vi "RIB Req - Fuse 5 Test.vi"(0 "Limits File Path":path, 5 "Results File Path":path, 11 "error in":errorcluster) -> (4 "Results Data Array":string[][](array[string]), 15 "error out":errorcluster)   [LabVIEW 2024]
doc: "Template test"
uses:
  <vilib>/addons/_JKI Toolkits/State Machine/_JKI_lib_State_Machine.llb/Select State(s)_err__jki_lib_state_machine.vi
  <vilib>/addons/_JKI Toolkits/State Machine/_JKI_lib_State_Machine.llb/Select State(s)_bool__jki_lib_state_machine.vi
  <vilib>/addons/_JKI Toolkits/State Machine/_JKI_lib_State_Machine.llb/Periodic Trigger__ogtk__JKI-SM__jki_lib_state_machine.vi
  <userlib>/_OpenG.lib/file/file.llb/Strip Path Extension - String__ogtk.vi
  <vilib>/Utility/file.llb/Read Delimited Spreadsheet (string).vi
  <userlib>/_OpenG.lib/file/file.llb/openg_file.lvlib
  <userlib>/_OpenG.lib/appcontrol/appcontrol.llb/openg_application_control.lvlib
  <userlib>/_OpenG.lib/time/time.llb/openg_time.lvlib
  <vilib>/Utility/file.llb/Write Delimited Spreadsheet (string).vi
panel:
  out "Timeout - Test 2":dbl(slide) scale=0.0..5.0
  out "State Test":bool
  in  "Fuse 5 State Error Test":string
  in  "Fuse 5 State Test":string
  in  "Read Start":string
  in  "Read Set":string
  out "Timeout - Test":dbl(slide) scale=0.0..5.0
  out "Fuse 5 Test":bool
  in  "Fuse 5 Error Test":string
  in  "Fuse 5 Test":string
  in  "connection ID":refnum<k16>
  in  "handle out":u64
  in  "Exit":bool
  # "Fuse 5 Test"
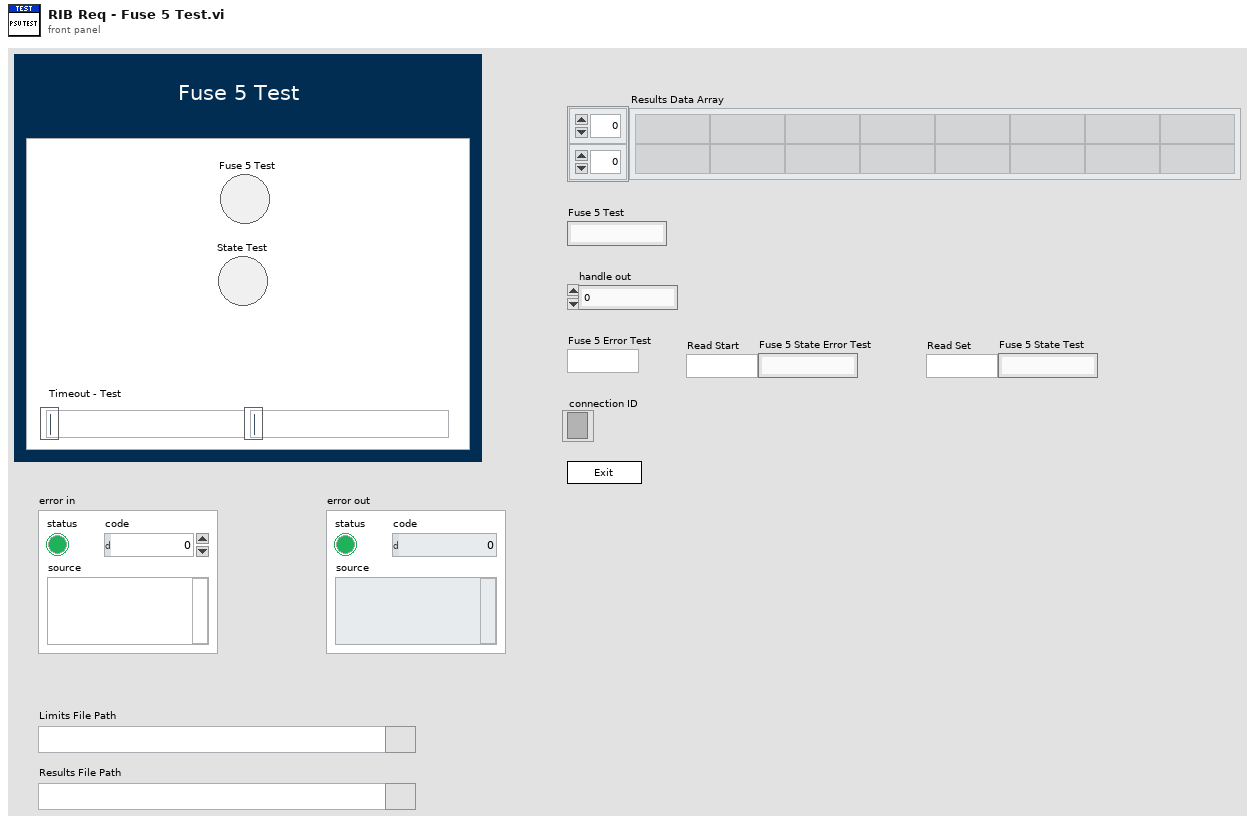
[diagram p1: front panel]
types:
  T1 = enum32{"Invalid", "Standard", "Closed", "Hidden", "Minimized", "Maximized"}
  T2 = enum32{"invalid app kind", "Development System", "Run Time System", "Student Edition", "Embedded LabVIEW", "Evaluation", "Custom"}
  T3 = typedef "FGV - Enum" = enum16{"Cleanup", "Get Data", "Simulator", "Open UDP", "Initialise DAQ", "Initialise I2C"}
  T4 = enum16{"Start Timer", "Get Time", "Pause", "Unpause"}
  T5 = cluster{"Core":cluster{"Current VI Reference":refnum<vi>, "Close Panel on Exit?":bool}, "Limits File Path":path, "Test Limits":string[][], "Results Data Array":string[][], "Results File Path":path, "Voltage":dbl, "connection ID":refnum<k16>, "handle out":u64, "Fuse 5 Test":string, "Fuse 5 Error Test":string, "Read Set":string, "Read Start ":string, "Fuse 5 State Test":string, "Fuse 5 State Error Test":string, "Monitor Test":bool}
  T6 = cluster{"Current VI Reference":refnum<vi>, "Close Panel on Exit?":bool}
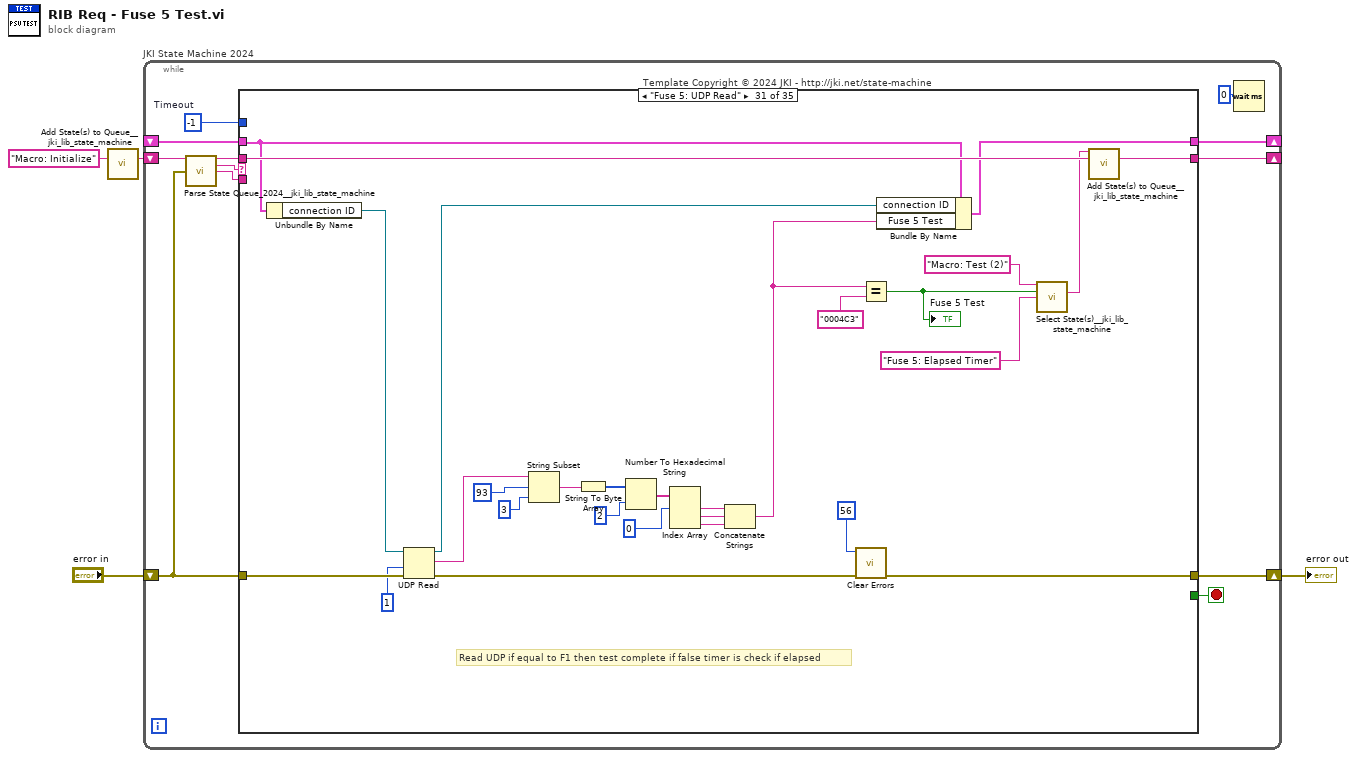
[diagram p0: block diagram]
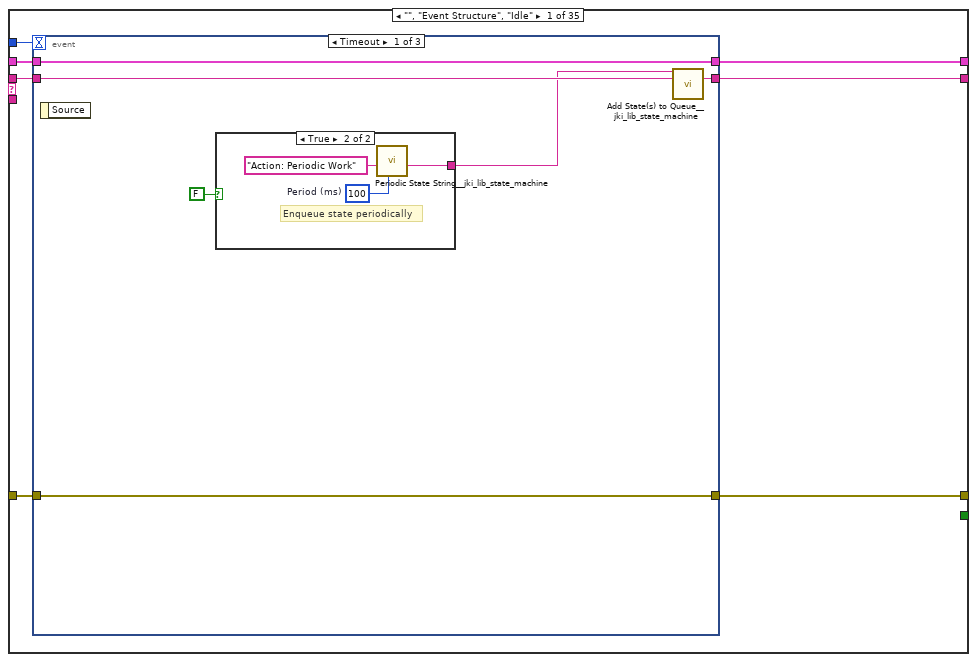
[diagram p2: hidden frame]
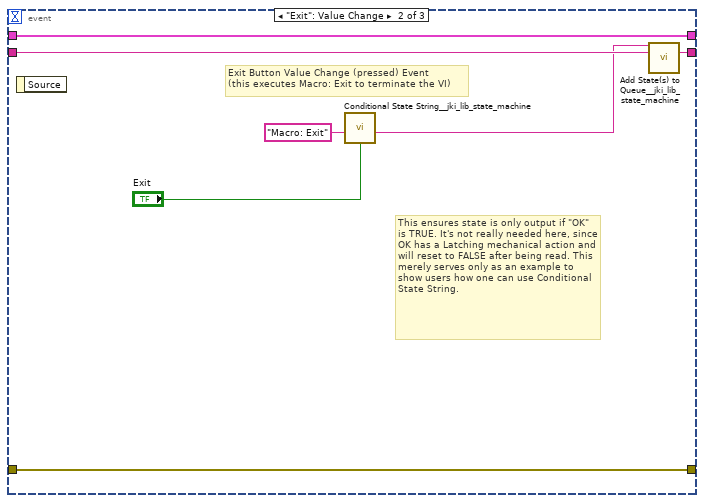
[diagram p4: hidden frame]
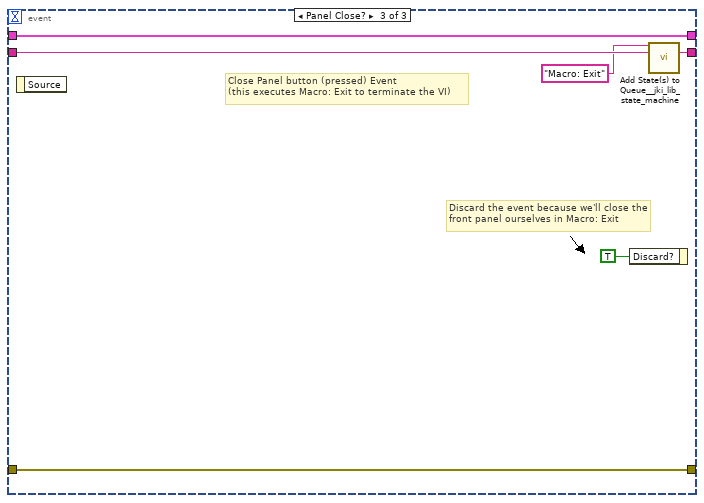
[diagram p5: hidden frame]
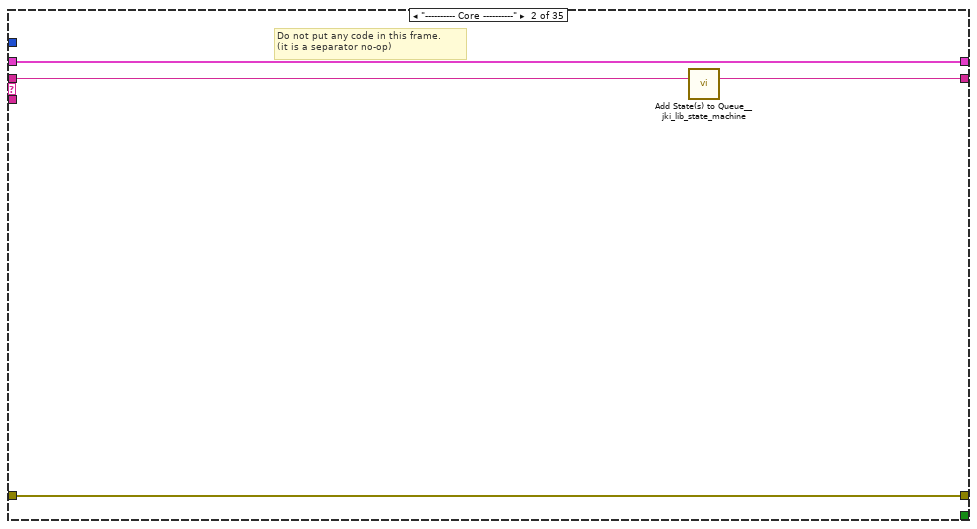
[diagram p6: hidden frame]
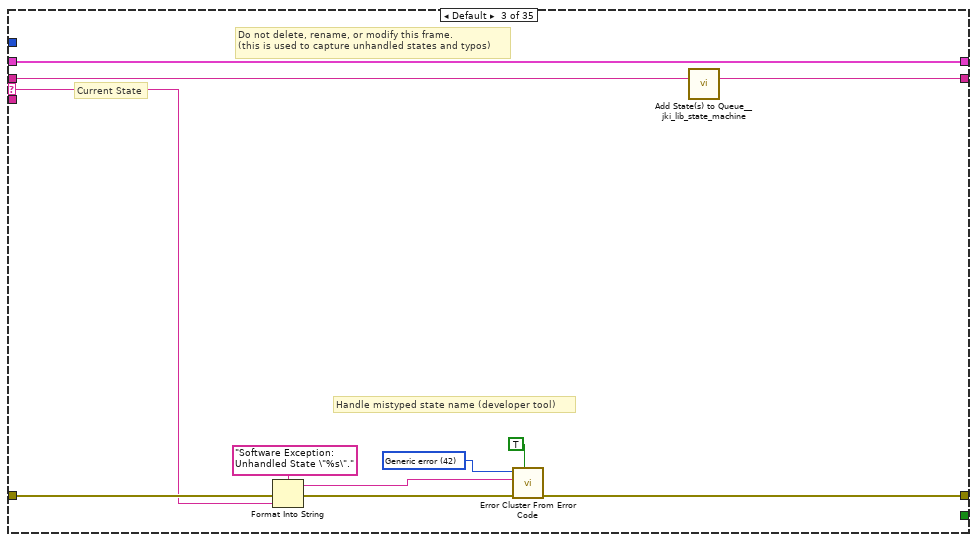
[diagram p7: hidden frame]
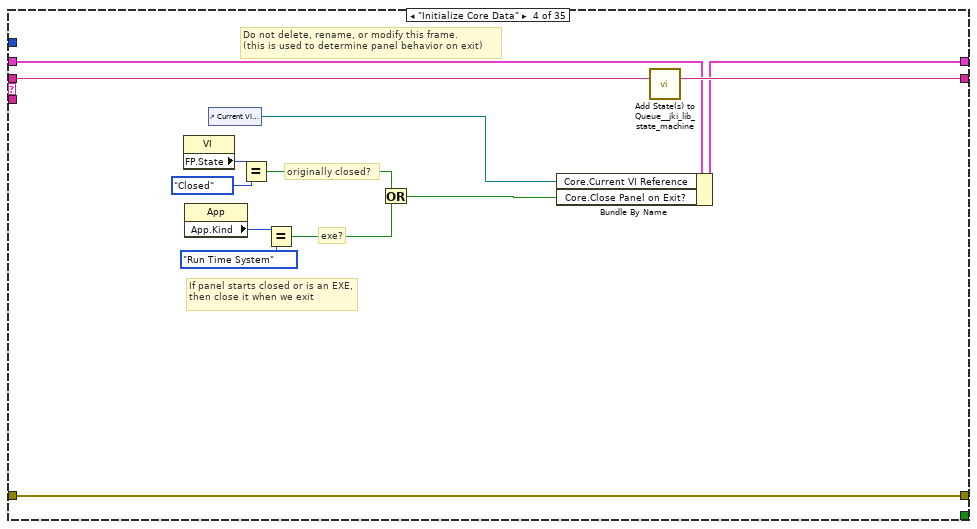
[diagram p8: hidden frame]
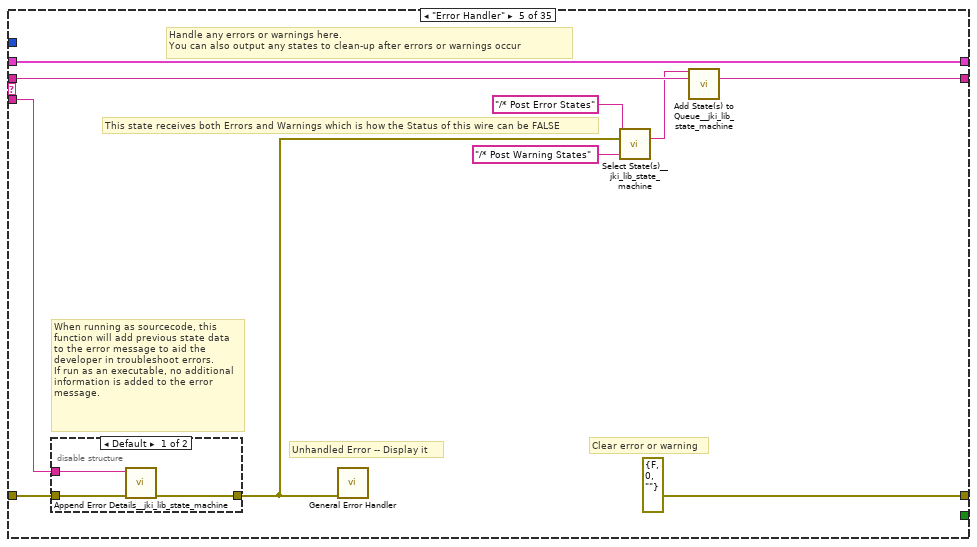
[diagram p9: hidden frame]
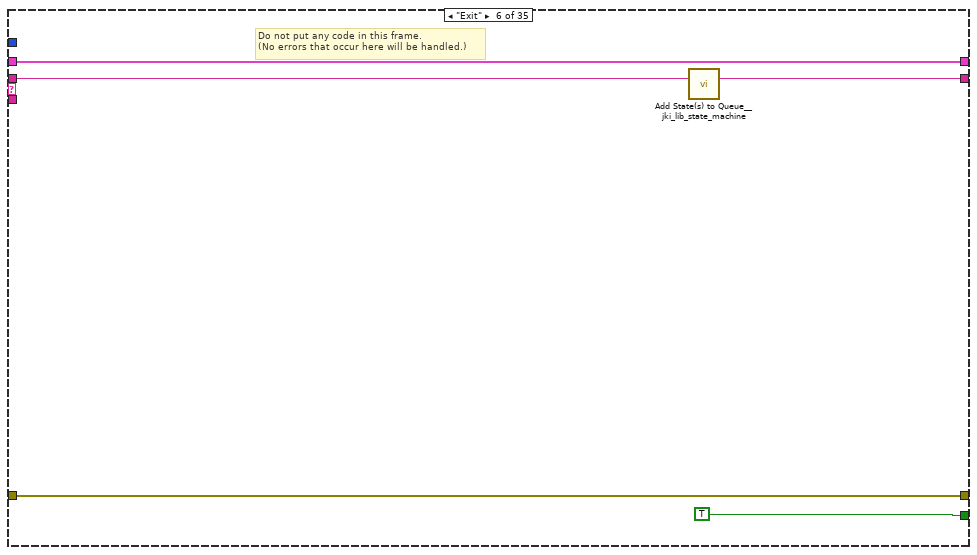
[diagram p11: hidden frame]
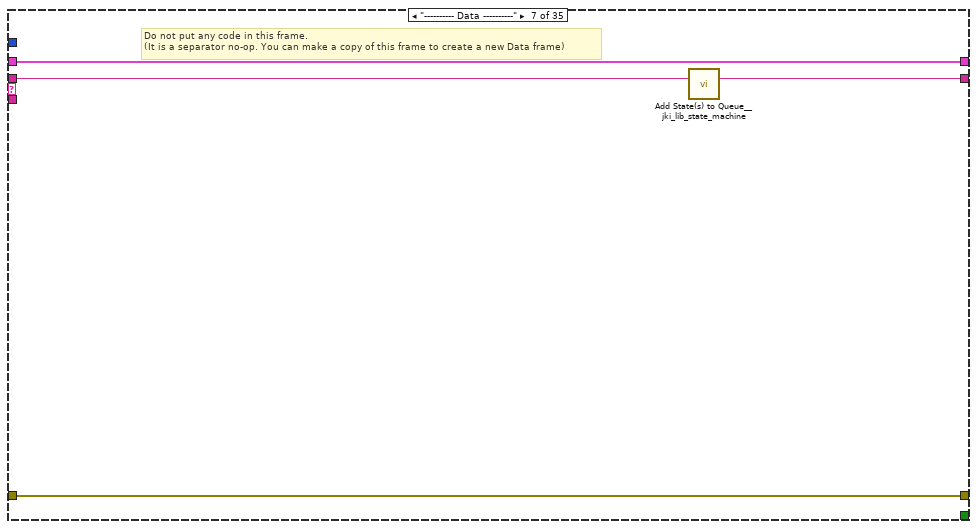
[diagram p12: hidden frame]
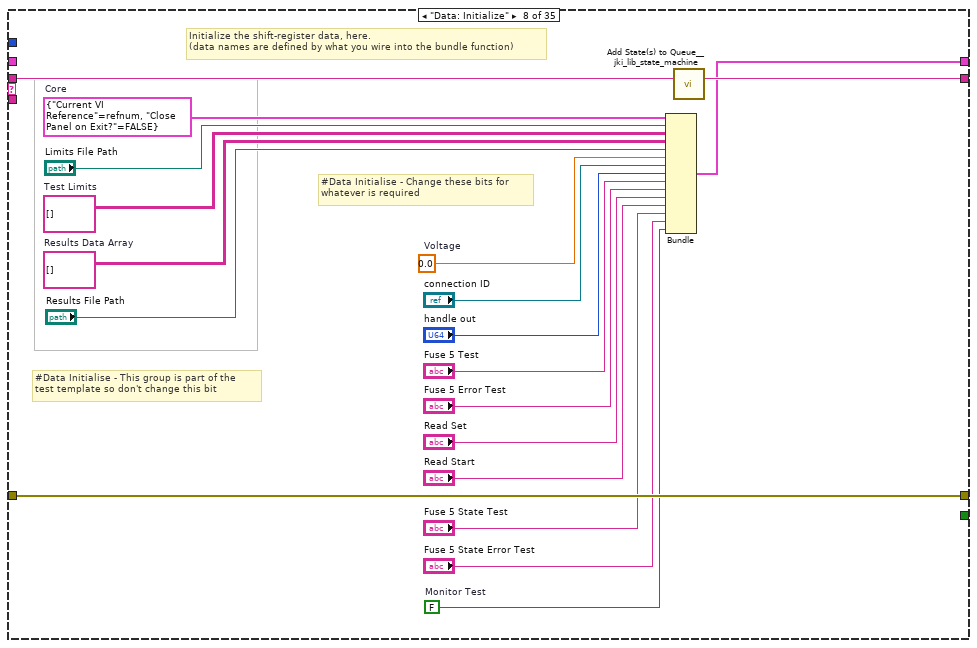
[diagram p13: hidden frame]
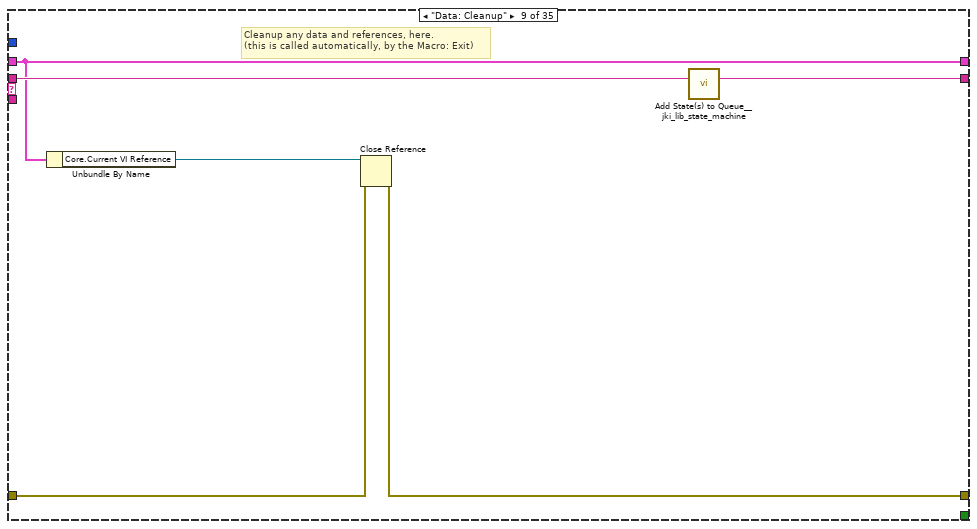
[diagram p14: hidden frame]
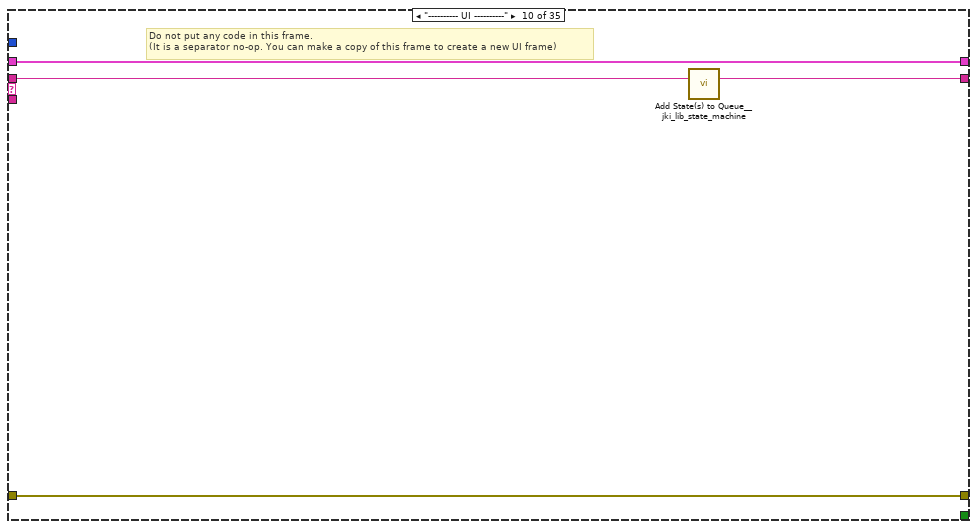
[diagram p15: hidden frame]
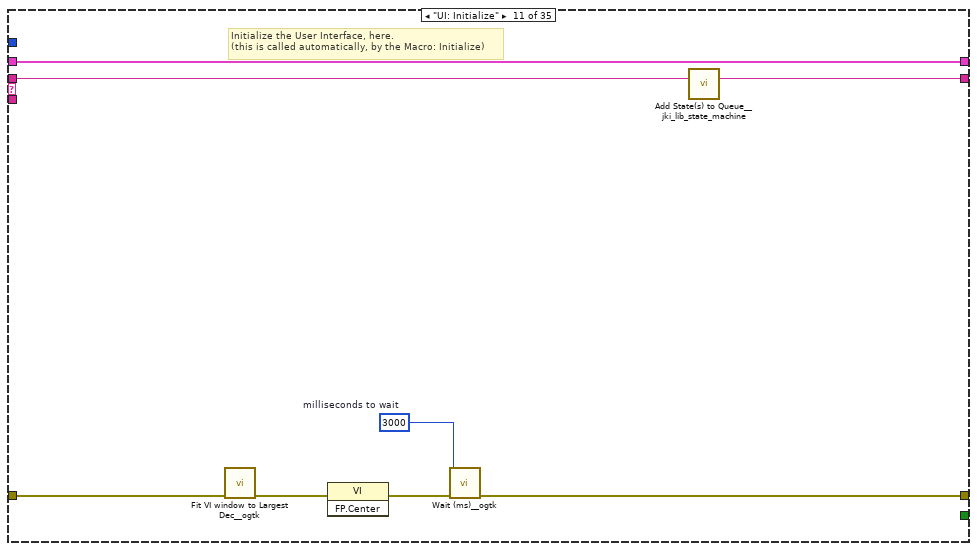
[diagram p16: hidden frame]
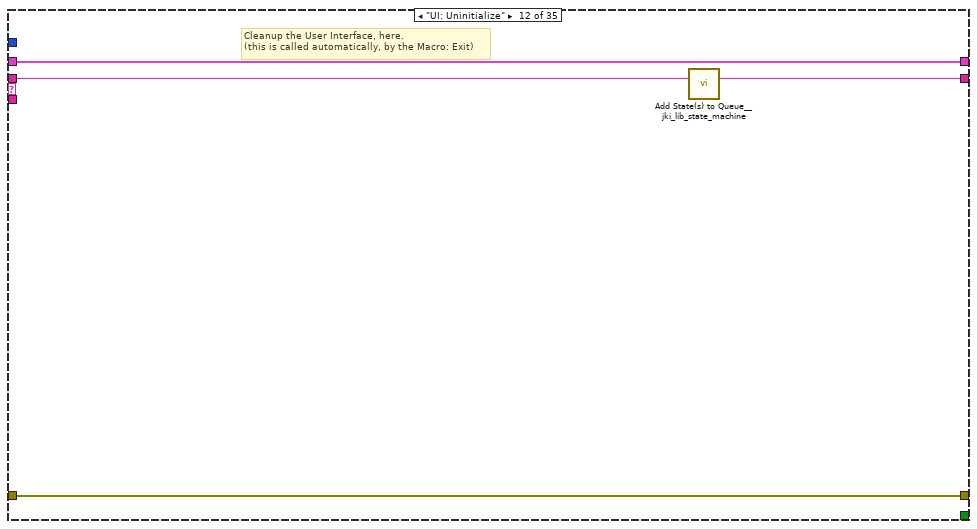
[diagram p17: hidden frame]
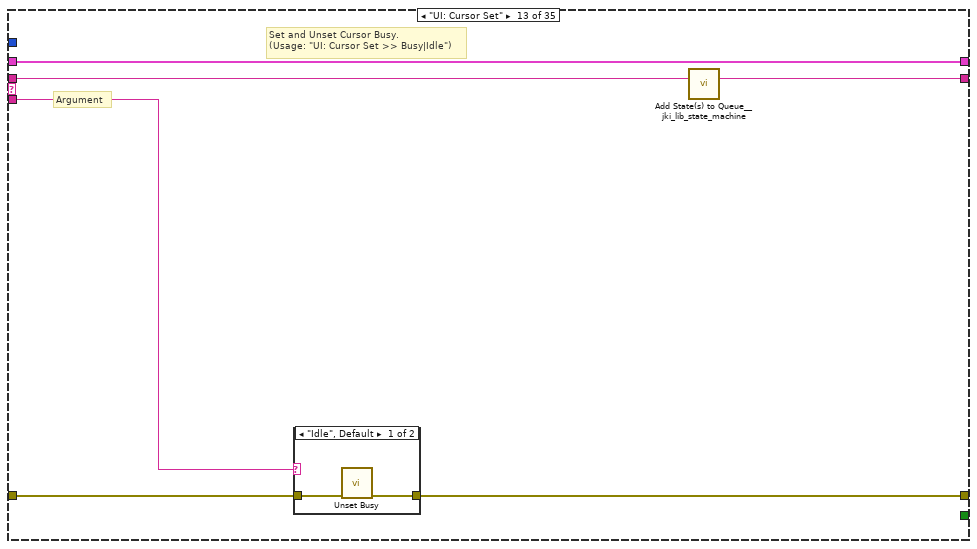
[diagram p18: hidden frame]
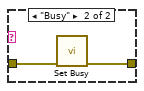
[diagram p19: hidden frame]
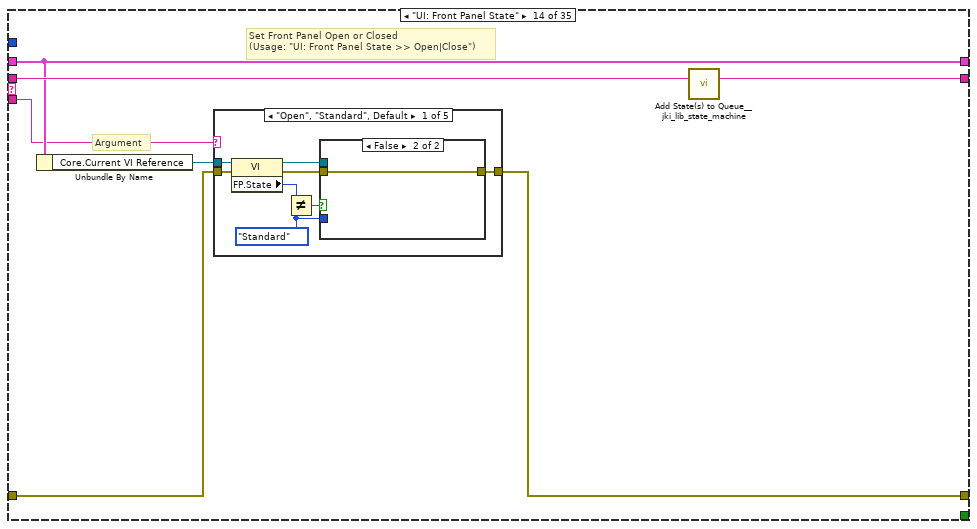
[diagram p20: hidden frame]
diagram:
  n1 = call <vilib>:"Add State(s) to Queue__jki_lib_state_machine.vi"("State(s) in (\"\")"="Macro: Initialize") -> ("States Out"=w4:string)  [unwired: 14 in]
  n2 = while "JKI State Machine 2024" {
    shift-right: [w9] -> _
    shift-left: _ -> [w8]
    shift-right: [w12] -> w1
    shift-left: "error in" -> [w6]
    shift-right: [w11] -> _
    shift-left: w4 -> [w13]
    stop <- w10 stop-if-true
    w7 = -1  # Timeout
    # "Template Copyright © 2024 JKI - http://jki.net/state-machine"
    n3 = call <vilib>:"Parse State Queue_2024__jki_lib_state_machine.vi"("State Queue"=w13, "Error In (no error)"=w6) -> ("Remaining States"=w15:string, "Current State"=w16:string, "Arguments"=w14:string)  [unwired: 11 in]
    n4 = case shown="\"Fuse 5: UDP Read\"" w16 {
      selector: w16 -> [_ _ w50 _ _ _ _ _ _ _ _ _ _ _ _ _ _ _ _ _ _ _ _ _ _ _ _ _ _ _ _ _ _ _ _]
      tunnel: w15 -> [w23 w49 w54 w73 w83 w92 w96 w115 w121 w125 w133 w137 w143 w154 w223 w228 w233 w238 w243 w252 w256 w269 w286 w299 w303 w312 w316 w325 w335 w344 w372 w384 w394 w418 w430]
      tunnel: w14 -> [_ _ _ _ w78 _ _ _ _ _ _ _ w138 w148 _ _ _ _ _ _ _ _ _ _ _ _ _ _ _ _ _ _ _ _ _]
      tunnel: w8 -> [w21 w46 w52 w66 w80 w90 w93 _ w116 w122 w131 w135 w141 w150 w220 w225 w230 w235 w240 w250 w253 w259 w278 w291 w300 w308 w313 w323 w333 w342 w356 w382 w392 w405 w428]
      tunnel: [w20 w47 w56 w70 errorcluster {"status"=FALSE, "code"=0, "source"=""} ("error out") w89 w94 w112 w117 w123 w129 w134 w139 w151 w221 w226 w231 w236 w241 w247 w254 w265 w283 w296 w301 w310 w314 w320 w326 w339 w354 w376 w385 w403 w422] -> w12
      tunnel: w6 -> [w17 w47 w55 w70 w79 w89 w94 w112 w118 w123 w130 w134 w140 w152 w221 w226 w231 w236 w241 w247 w254 w264 w282 w295 w301 w309 w314 w321 w327 w340 w357 w377 w386 w399 w423]
      tunnel: [w22 w48 w53 w72 w82 w91 w95 w114 w120 w124 w132 w136 w142 w153 w222 w227 w232 w237 w242 w251 w255 w268 w285 w298 w302 w311 w315 w324 w334 w343 w371 w383 w393 w417 w429] -> w11
      tunnel: [_ _ _ _ _ TRUE _ _ _ _ _ _ _ _ _ _ _ _ _ _ _ _ _ _ _ _ _ _ _ _ _ _ _ _ _] -> w10
      tunnel: [w19 w46 w52 w71 w80 w90 w93 w113 w116 w122 w131 w135 w141 w150 w220 w225 w230 w235 w240 w250 w253 w258 w277 w290 w300 w308 w313 w322 w333 w341 w370 w382 w392 w416 w428] -> w9
      tunnel: w7 -> [w18 _ _ _ _ _ _ _ _ _ _ _ _ _ _ _ _ _ _ _ _ _ _ _ _ _ _ _ _ _ _ _ _ _ _]
      frame "", "Event Structure", "Idle" {
        n5 = event shown="[0] Timeout" {
          selector: _ -> [_ _ _]
          dyn-events: _ -> [_ _ _]
          timeout: w18 -> [_ _ _]
          tunnel: w23 -> [w29 w39 w45]
          tunnel: [w28 w38 w44] -> w22
          tunnel: w21 -> [w26 w36 w42]
          tunnel: [w27 w37 w43] -> w20
          tunnel: w17 -> [w27 w37 w43]
          tunnel: [w26 w36 w42] -> w19
          event Timeout {
            n6 = event-data() -> ()  [unwired: 1 in, 1 out]
            n7 = case shown="True" FALSE {
              tunnel: [_ w32] -> w25
              frame False {
              }
              frame True {
                w30 = u32 100  # Period (ms)
                # "Enqueue state periodically"
                n8 = call <vilib>:"Periodic State String__jki_lib_state_machine.vi"("Period (ms)"=w30, "State"="Action: Periodic Work") -> ("State Out"=w32:string)  [unwired: 9 in]
              }
            }
            n9 = call <vilib>:"Add State(s) to Queue__jki_lib_state_machine.vi"("State(s) in Front (\"\")"=w25, "State(s) in (\"\")"=w29) -> ("States Out"=w28:string)  [unwired: 13 in]
          }
          event "Exit": Value Change {
            # "This ensures state is only output if \"OK\" is TRUE. It's not really needed here, since OK has a Latching mechanical action and will reset to FALSE after being read. This merely serves only as an example to show users how one can use Conditional State String."
            # "Exit Button Value Change (pressed) Event\n(this executes Macro: Exit to terminate the VI)"
            n10 = event-data() -> ()  [unwired: 1 in, 1 out]
            n11 = call <vilib>:"Conditional State String__jki_lib_state_machine.vi"("Do State(s)?"="Exit", "State"="Macro: Exit") -> ("State Out"=w33:string)  [unwired: 7 in]
            n12 = call <vilib>:"Add State(s) to Queue__jki_lib_state_machine.vi"("State(s) in Front (\"\")"=w33, "State(s) in (\"\")"=w39) -> ("States Out"=w38:string)  [unwired: 13 in]
          }
          event Panel Close? {
            # "Discard the event because we'll close the front panel ourselves in Macro: Exit"
            # "Close Panel button (pressed) Event\n(this executes Macro: Exit to terminate the VI)"
            n13 = event-data() -> ()  [unwired: 1 in, 1 out]
            n14 = event-data("Discard?"=TRUE) -> ()  [unwired: 1 in, 1 out]
            n15 = call <vilib>:"Add State(s) to Queue__jki_lib_state_machine.vi"("State(s) in Front (\"\")"="Macro: Exit", "State(s) in (\"\")"=w45) -> ("States Out"=w44:string)  [unwired: 13 in]
          }
        }
      }
      frame "---------- Core ----------" {
        # "Do not put any code in this frame.\n(it is a separator no-op)"
        n16 = call <vilib>:"Add State(s) to Queue__jki_lib_state_machine.vi"("State(s) in (\"\")"=w49) -> ("States Out"=w48:string)  [unwired: 14 in]
      }
      frame Default {
        w59 = 42 items=["No error", "Argument error", "Memory is full", "Out of zone", "End of file", "File already open", "Generic file I/O error", "File not found", "File permission error", "Disk is full", "Duplicate path", "Too many files open", "System feature not enabled", "Resource file not found", "Cannot add resource", "Resource not found", "Image not found", "Image memory error", "Pen does not exist", "Config type invalid", "Config token not found", "Config parse error", "Config memory error", "Bad external code format", "Bad external code offset", "External code not present", "Null window", "Destroy window error", "Null menu", "Print aborted", "Bad print record", "Print driver error", "Windows error during printing", "Memory error during printing", "Print dialog error", "Generic print error", "Invalid device refnum", "Device not found", "Device parameter error", "Device unit error", "Cannot open device", "Device call aborted", "Generic error", "Cancelled by user", "Object ID too low", "Object ID too high", "Object not in heap", "Unknown heap", "Unknown object (invalid DefProc)", "Unknown object (DefProc not in table)", "Message out of range", "Invalid (null) method", "Unknown message", "Manager call not supported", "Bad address", "Network operation in progress", "Network operation timed out", "Connection is busy", "Network attribute not supported", "Network error", "Address in use", "System out of memory", "Connection aborted", "Connection refused", "Not connected", "Already connected", "Connection closed", "Initialization error (interapplication manager)", "Bad occurrence", "Wait on unbound occurrence handler", "Occurrence queue overflow", "Datalog type conflict", "Unused", "Unrecognized type (interapplication manager)", "Memory corrupt", "Failed to make temporary DLL", "Old CIN version", "Drag socket not found", "Failed to load drop-object", "Failed to register OLE object", "Failed to release OLE object", "Format specifier type mismatch", "Unknown format specifier", "Too few format specifiers", "Too many format specifiers", "Scan failed", "Newer CIN version", "Error converting to variant", "Runtime menu error", "Password tampered", "Variant attribute not found", "Incompatible variant data type", "Event data is not available", "Event Store is not present", "Occurrence is not found", "Event Queue is not created", "Event info is not available", "Refnum passed is NULL", "Error retrieving Class GUID", "Error retrieving CoClass GUID", "Error retrieving TypeLib GUID.", "Bad built application magic bytes.", "Specific driver is different from the specific driver associated with the Logical Name.", "There is no session opened to the class driver.", "Max Error", "MAX - Error with config objects", "MAX - Error loading configuration", "MAX - Group not supported"]
        # "Current State"
        # "Do not delete, rename, or modify this frame.\n(this is used to capture unhandled states and typos)"
        # "Handle mistyped state name (developer tool)"
        n17 = Format Into String(format string="Software Exception: Unhandled State \"%s\"." ("message"), error in=w55, w50) -> (resulting string=w58:string, error out=w57:errorcluster)  [unwired: 1 in]
        n18 = call <vilib>:"Error Cluster From Error Code.vi"("show call chain? (False)"=TRUE, "error in (no error)"=w57, "error message (\"\")"=w58, "error code (0)"=w59) -> ("error out"=w56:errorcluster)  [unwired: 5 in]
        n19 = call <vilib>:"Add State(s) to Queue__jki_lib_state_machine.vi"("State(s) in (\"\")"=w54) -> ("States Out"=w53:string)  [unwired: 14 in]
      }
      frame "Initialize Core Data" {
        # "Do not delete, rename, or modify this frame.\n(this is used to determine panel behavior on exit)"
        # "originally closed?"
        # "exe?"
        # "If panel starts closed or is an EXE, then close it when we exit"
        n20 = property class="VI"() -> ("FP.State"=w63:T1)  [unwired: 2 in, 2 out]
        n21 = property class="App"() -> ("App.Kind"=w69:T2)  [unwired: 2 in, 2 out]
        n22 = control-ref of="Current VI Reference"() -> (w64:refnum<vi>)
        n23 = Equal?(x=w63, y=T1."Closed" ("Front Panel Window:State")) -> (x = y?=w61:bool)
        n24 = Equal?(x=w69, y=T2."Run Time System" ("Application:Kind")) -> (x = y?=w67:bool)
        n25 = Or(x=w61, y=w67) -> (x .or. y?=w65:bool)
        n26 = Bundle By Name(cluster=w66, "Core.Current VI Reference"=w64, "Core.Close Panel on Exit?"=w65) -> (w71:T5)
        n27 = call <vilib>:"Add State(s) to Queue__jki_lib_state_machine.vi"("State(s) in (\"\")"=w73) -> ("States Out"=w72:string)  [unwired: 14 in]
      }
      frame "Error Handler" {
        # "When running as sourcecode, this function will add previous state data to the error message to aid the developer in troubleshoot errors.\nIf run as an executable, no additional information is added to the error message."
        # "This state receives both Errors and Warnings which is how the Status of this wire can be FALSE"
        # "Unhandled Error -- Display it"
        # "Handle any errors or warnings here.\nYou can also output any states to clean-up after errors or warnings occur"
        # "Clear error or warning"
        n28 = disable-structure shown="Default" {
          disable-tunnel: w79 -> [w86 w87]
          disable-tunnel: w78 -> [w85 _]
          disable-tunnel: [w84 w87] -> w77
          frame condition #0 (active) {
            n29 = call <vilib>:"Append Error Details__jki_lib_state_machine.vi"("error in (no error)"=w86, "Previous State and Argument(s)"=w85) -> ("error out"=w84:errorcluster)  [unwired: 9 in]
          }
          frame condition #1 {
          }
        }
        n30 = call <vilib>:"General Error Handler.vi"("error in (no error)"=w77) -> ()  [unwired: 10 in, 5 out]
        n31 = call-poly <vilib>:"Select State(s)__jki_lib_state_machine.vi"("State(s) if True (\"\")"="/* Post Error States", "Select"=w77, "State(s) if False (\"\")"="/* Post Warning States") -> ("States Out"=w75:string)  [unwired: 12 in]
        n32 = call <vilib>:"Add State(s) to Queue__jki_lib_state_machine.vi"("State(s) in Front (\"\")"=w75, "State(s) in (\"\")"=w83) -> ("States Out"=w82:string)  [unwired: 13 in]
      }
      frame "Exit" {
        # "Do not put any code in this frame.\n(No errors that occur here will be handled.)"
        n33 = call <vilib>:"Add State(s) to Queue__jki_lib_state_machine.vi"("State(s) in (\"\")"=w92) -> ("States Out"=w91:string)  [unwired: 14 in]
      }
      frame "---------- Data ----------" {
        # "Do not put any code in this frame.\n(It is a separator no-op. You can make a copy of this frame to create a new Data frame)"
        n34 = call <vilib>:"Add State(s) to Queue__jki_lib_state_machine.vi"("State(s) in (\"\")"=w96) -> ("States Out"=w95:string)  [unwired: 14 in]
      }
      frame "Data: Initialize" {
        w97 = FALSE  # Monitor Test
        w106 = 0.0  # Voltage
        w108 = string[][] []  # Results Data Array
        w109 = string[][] []  # Test Limits
        w111 = T6 {"Current VI Reference"=refnum, "Close Panel on Exit?"=FALSE}  # Core
        # "#Data Initialise - Change these bits for\nwhatever is required"
        # "#Data Initialise - This group is part of the\ntest template so don't change this bit"
        # "Initialize the shift-register data, here.\n(data names are defined by what you wire into the bundle function)"
        n35 = Bundle("Core"=w111, "Limits File Path"="Limits File Path", "Test Limits"=w109, "Results Data Array"=w108, "Results File Path"="Results File Path", "Voltage"=w106, "connection ID"="connection ID", "handle out"="handle out", "Fuse 5 Test"="Fuse 5 Test", "Fuse 5 Error Test"="Fuse 5 Error Test", "Read Set"="Read Set", "Read Start"="Read Start", "Fuse 5 State Test"="Fuse 5 State Test", "Fuse 5 State Error Test"="Fuse 5 State Error Test", "Monitor Test"=w97) -> (w113:T5)  [unwired: 1 in]
        n36 = call <vilib>:"Add State(s) to Queue__jki_lib_state_machine.vi"("State(s) in (\"\")"=w115) -> ("States Out"=w114:string)  [unwired: 14 in]
      }
      frame "Data: Cleanup" {
        # "Cleanup any data and references, here.\n(this is called automatically, by the Macro: Exit)"
        n37 = Unbundle By Name(w116) -> ("Core.Current VI Reference"=w119:refnum<vi>)
        n38 = Close Reference(reference=w119, error in (no error)=w118) -> (error out=w117:errorcluster)
        n39 = call <vilib>:"Add State(s) to Queue__jki_lib_state_machine.vi"("State(s) in (\"\")"=w121) -> ("States Out"=w120:string)  [unwired: 14 in]
      }
      frame "---------- UI ----------" {
        # "Do not put any code in this frame.\n(It is a separator no-op. You can make a copy of this frame to create a new UI frame)"
        n40 = call <vilib>:"Add State(s) to Queue__jki_lib_state_machine.vi"("State(s) in (\"\")"=w125) -> ("States Out"=w124:string)  [unwired: 14 in]
      }
      frame "UI: Initialize" {
        w128 = u32 3000  # milliseconds to wait
        # "Initialize the User Interface, here.\n(this is called automatically, by the Macro: Initialize)"
        n41 = call <userlib>:"Fit VI window to Largest Dec__ogtk.vi"("error in (no error)"=w130) -> ("error out"=w126:errorcluster)  [unwired: 5 in, 1 out]
        n42 = invoke class="VI" method="FP.Center"(error in=w126) -> (error out=w127:errorcluster)  [unwired: 2 in, 2 out]
        n43 = call <userlib>:"Wait (ms)__ogtk.vi"("error in (no error)"=w127, "milliseconds to wait"=w128) -> ("error out"=w129:errorcluster)  [unwired: 8 in, 1 out]
        n44 = call <vilib>:"Add State(s) to Queue__jki_lib_state_machine.vi"("State(s) in (\"\")"=w133) -> ("States Out"=w132:string)  [unwired: 14 in]
      }
      frame "UI: Uninitialize" {
        # "Cleanup the User Interface, here.\n(this is called automatically, by the Macro: Exit)"
        n45 = call <vilib>:"Add State(s) to Queue__jki_lib_state_machine.vi"("State(s) in (\"\")"=w137) -> ("States Out"=w136:string)  [unwired: 14 in]
      }
      frame "UI: Cursor Set" {
        # "Argument"
        # "Set and Unset Cursor Busy.\n(Usage: \"UI: Cursor Set >> Busy|Idle\")"
        n46 = case shown="\"Idle\", Default" w138 {
          tunnel: w140 -> [w145 w147]
          tunnel: [w144 w146] -> w139
          frame "Idle", Default {
            n47 = call <vilib>:"Unset Busy.vi"("error in (no error)"=w145) -> ("error out"=w144:errorcluster)  [unwired: 10 in]
          }
          frame "Busy" {
            n48 = call <vilib>:"Set Busy.vi"("error in (no error)"=w147) -> ("error out"=w146:errorcluster)  [unwired: 9 in, 1 out]
          }
        }
        n49 = call <vilib>:"Add State(s) to Queue__jki_lib_state_machine.vi"("State(s) in (\"\")"=w143) -> ("States Out"=w142:string)  [unwired: 14 in]
      }
      frame "UI: Front Panel State" {
        # "Argument"
        # "Set Front Panel Open or Closed\n(Usage: \"UI: Front Panel State >> Open|Close\")"
        n50 = Unbundle By Name(w150) -> ("Core.Current VI Reference"=w149:refnum<vi>)
        n51 = case shown="\"Open\", \"Standard\", Default" w148 {
          tunnel: w152 -> [w160 w175 w186 w199 w212]
          tunnel: [w162 w176 w188 w201 w214] -> w151
          tunnel: w149 -> [w161 w173 w187 w200 w213]
          frame "Open", "Standard", Default {
            w155 = T1."Standard" ("State")
            n52 = property class="VI"(reference=w161, error in=w160) -> (reference out=w158:refnum<vi>, error out=w159:errorcluster, "FP.State"=w157:T1)
            n53 = Not Equal?(x=w157, y=w155) -> (x != y?=w156:bool)
            n54 = case shown="False" w156 {
              tunnel: [w166 w168] -> w162
              tunnel: w159 -> [w165 w168]
              tunnel: w158 -> [w164 _]
              tunnel: w155 -> [w163 _]
              frame True {
                n55 = invoke class="VI" method="FP.Open"(reference=w164, error in=w165, "Activate"=TRUE, "State"=w163) -> (error out=w166:errorcluster)  [unwired: 1 in, 4 out]
              }
              frame False {
              }
            }
          }
          frame "Close", "Closed" {
            n56 = property class="VI"(reference=w173, error in=w175) -> (reference out=w172:refnum<vi>, error out=w174:errorcluster, "FP.State"=w170:T1)
            n57 = Not Equal?(x=w170, y=T1."Closed" ("Front Panel Window:State")) -> (x != y?=w169:bool)
            n58 = case shown="True" w169 {
              tunnel: [w177 w180] -> w176
              tunnel: w174 -> [w177 w179]
              tunnel: w172 -> [_ w178]
              frame False {
              }
              frame True {
                n59 = invoke class="VI" method="FP.Close"(reference=w178, error in=w179) -> (error out=w180:errorcluster)  [unwired: 1 in, 2 out]
              }
            }
          }
          frame "Hidden", "Hide" {
            w181 = T1."Hidden" ("State")
            n60 = property class="VI"(reference=w187, error in=w186) -> (reference out=w184:refnum<vi>, error out=w185:errorcluster, "FP.State"=w183:T1)
            n61 = Not Equal?(x=w183, y=w181) -> (x != y?=w182:bool)
            n62 = case shown="True" w182 {
              tunnel: [w192 w193] -> w188
              tunnel: w185 -> [w191 w193]
              tunnel: w184 -> [w190 _]
              tunnel: w181 -> [w189 _]
              frame True {
                n63 = invoke class="VI" method="FP.Open"(reference=w190, error in=w191, "State"=w189) -> (error out=w192:errorcluster)  [unwired: 2 in, 4 out]
              }
              frame False {
              }
            }
          }
          frame "Minimize", "Minimized" {
            w194 = T1."Minimized" ("State")
            n64 = property class="VI"(reference=w200, error in=w199) -> (reference out=w197:refnum<vi>, error out=w198:errorcluster, "FP.State"=w196:T1)
            n65 = Not Equal?(x=w196, y=w194) -> (x != y?=w195:bool)
            n66 = case shown="True" w195 {
              tunnel: [w205 w206] -> w201
              tunnel: w198 -> [w204 w206]
              tunnel: w197 -> [w203 _]
              tunnel: w194 -> [w202 _]
              frame True {
                n67 = invoke class="VI" method="FP.Open"(reference=w203, error in=w204, "State"=w202) -> (error out=w205:errorcluster)  [unwired: 2 in, 4 out]
              }
              frame False {
              }
            }
          }
          frame "Maximize", "Maximized" {
            w207 = T1."Maximized" ("State")
            n68 = property class="VI"(reference=w213, error in=w212) -> (reference out=w210:refnum<vi>, error out=w211:errorcluster, "FP.State"=w209:T1)
            n69 = Not Equal?(x=w209, y=w207) -> (x != y?=w208:bool)
            n70 = case shown="True" w208 {
              tunnel: [w218 w219] -> w214
              tunnel: w211 -> [w217 w219]
              tunnel: w210 -> [w216 _]
              tunnel: w207 -> [w215 _]
              frame True {
                n71 = invoke class="VI" method="FP.Open"(reference=w216, error in=w217, "State"=w215) -> (error out=w218:errorcluster)  [unwired: 2 in, 4 out]
              }
              frame False {
              }
            }
          }
        }
        n72 = call <vilib>:"Add State(s) to Queue__jki_lib_state_machine.vi"("State(s) in (\"\")"=w154) -> ("States Out"=w153:string)  [unwired: 14 in]
      }
      frame "---------- Macro ----------" {
        # "Do not put any code in this frame.\n(It is a separator no-op. You can make a copy of this frame to create a new Macro frame)"
        n73 = call <vilib>:"Add State(s) to Queue__jki_lib_state_machine.vi"("State(s) in (\"\")"=w223) -> ("States Out"=w222:string)  [unwired: 14 in]
      }
      frame "Macro: Initialize" {
        # "Initialization Macro\n(This is called once, when the VI starts)"
        n74 = call <vilib>:"Add State(s) to Queue__jki_lib_state_machine.vi"("State(s) in Front (\"\")"="Data: Initialize\nInitialize Core Data\nUI: Initialize\nUI: Front Panel State >> Open\nFuse 5: Initialise\nMacro: Test", "State(s) in (\"\")"=w228) -> ("States Out"=w227:string)  [unwired: 13 in]
      }
      frame "Macro: Test" {
        # "#Test Macro - Add the sequence \nfor measurments and limits testing here"
        n75 = call <vilib>:"Add State(s) to Queue__jki_lib_state_machine.vi"("State(s) in Front (\"\")"="Limits Test: Read Limits File\nFuse 5: Initialise\nFuse 5: Start Timer\nFuse 5: I2C Measurment\nFuse 5: UDP Read", "State(s) in (\"\")"=w233) -> ("States Out"=w232:string)  [unwired: 13 in]
      }
      frame "Macro: Test (2)" {
        # "#Test Macro - Add the sequence \nfor measurments and limits testing here"
        n76 = call <vilib>:"Add State(s) to Queue__jki_lib_state_machine.vi"("State(s) in Front (\"\")"="Fuse 5: Start Timer (State)\nFuse 5: UDP Read (State)", "State(s) in (\"\")"=w238) -> ("States Out"=w237:string)  [unwired: 13 in]
      }
      frame "Macro: Limits" {
        # "Do not put any code in this frame.\n(It is a separator no-op. You can make a copy of this frame to create a new Macro frame)"
        n77 = call <vilib>:"Add State(s) to Queue__jki_lib_state_machine.vi"("State(s) in Front (\"\")"="Limits Test: Fuse 5 Test\nLimits Test: Fuse 5 State Test\nResults Data: Write Results Data\nMacro: Exit", "State(s) in (\"\")"=w243) -> ("States Out"=w242:string)  [unwired: 13 in]
      }
      frame "Macro: Exit" {
        # "Exit Macro\n(This is called once, when the VI exits)"
        n78 = Unbundle By Name(w250) -> ("Core.Close Panel on Exit?"=w245:bool)
        n79 = call <vilib>:"Conditional State String__jki_lib_state_machine.vi"("Do State(s)?"=w245, "State"="UI: Front Panel State >> Close") -> ("State Out"=w244:string)  [unwired: 7 in]
        n80 = call <vilib>:"Add State(s) to Queue__jki_lib_state_machine.vi"("State(s) in (\"\")"=w244, "State(s) at Back (\"\")"="UI: Uninitialize\nData: Cleanup\nExit") -> ("States Out"=w248:string)  [unwired: 13 in]
        n81 = call <vilib>:"Add State(s) to Queue__jki_lib_state_machine.vi"("State(s) in Front (\"\")"=w248, "State(s) in (\"\")"=w252) -> ("States Out"=w251:string)  [unwired: 13 in]
      }
      frame "---------- Limits Test ----------" {
        # "Template Separator\n(You can make a copy of, or modify, this frame)"
        n82 = call <vilib>:"Add State(s) to Queue__jki_lib_state_machine.vi"("State(s) in (\"\")"=w256) -> ("States Out"=w255:string)  [unwired: 14 in]
      }
      frame "Limits Test: Read Limits File" {
        w262 = ","  # delimiter (\t)
        n83 = Unbundle By Name(w259) -> ("Limits File Path"=w263:path)
        n84 = Current VI's Path "Test Case Path"() -> (path=w267:path)
        n85 = call-poly <vilib>:"Read Delimited Spreadsheet.vi"("file path (dialog if empty)"=w263, "error in (no error)"=w264, "delimiter (\\t)"=w262) -> ("all rows"=w260:string[][], "error out"=w265:errorcluster)  [unwired: 7 in, 4 out]
        n86 = Strip Path(path=w267) -> (name=w266:string)  [unwired: 1 out]
        n87 = call-poly <userlib>:"Strip Path Extension__ogtk.vi"("path"=w266) -> ("root"=w261:string)  [unwired: 1 out]
        n88 = for {
          tunnel: w261 -> [w273]
          tunnel: w260 -> [w271] mode=indexing
          tunnel: [w271] -> w257 mode=indexing if=w270
          n89 = Index Array(array=w271) -> (element=w272:string)  [unwired: 1 in]
          n90 = Equal?(x=w273, y=w272) -> (x = y?=w270:bool)
        }
        n91 = Bundle By Name(cluster=w259, "Test Limits"=w257) -> (w258:T5)
        n92 = call <vilib>:"Add State(s) to Queue__jki_lib_state_machine.vi"("State(s) in (\"\")"=w269) -> ("States Out"=w268:string)  [unwired: 14 in]
      }
      frame "Limits Test: Fuse 5 Test" {
        w279 = "Fuse 5 Test"  # Sub Test Name
        # "Equal to F1?"
        # "#Limits Testing - Add the sub test name for\ntest included in limits file"
        n93 = Unbundle By Name(w278) -> ("Results Data Array"=w276:string[][])
        n94 = Unbundle By Name(w278) -> ("Test Limits"=w280:string[][], "Fuse 5 Test"=w284:string)
        n95 = To Variant(anything=w284) -> (Variant=w281:variant)
        n96 = call "Process Results.vi"("error in (no error)"=w282, "Measurement"=w281, "Test Limits"=w280, "Sub Test Name"=w279) -> ("error out"=w283:errorcluster, "Results Data"=w275:string[])  [unwired: 6 in]
        n97 = Build Array (concatenate)(w276, w275) -> (w274:string[][])
        n98 = Bundle By Name(cluster=w278, "Results Data Array"=w274) -> (w277:T5)
        n99 = call <vilib>:"Add State(s) to Queue__jki_lib_state_machine.vi"("State(s) in (\"\")"=w286) -> ("States Out"=w285:string)  [unwired: 14 in]
      }
      frame "Limits Test: Fuse 5 State Test" {
        w292 = "Fuse 5 State Test"  # Sub Test Name
        # "Equal to F1?"
        # "#Limits Testing - Add the sub test name for\ntest included in limits file"
        n100 = Unbundle By Name(w291) -> ("Test Limits"=w293:string[][], "Fuse 5 State Test"=w297:string)
        n101 = Unbundle By Name(w291) -> ("Results Data Array"=w289:string[][])
        n102 = To Variant(anything=w297) -> (Variant=w294:variant)
        n103 = call "Process Results.vi"("error in (no error)"=w295, "Measurement"=w294, "Test Limits"=w293, "Sub Test Name"=w292) -> ("error out"=w296:errorcluster, "Results Data"=w288:string[])  [unwired: 6 in]
        n104 = Build Array (concatenate)(w289, w288) -> (w287:string[][])
        n105 = Bundle By Name(cluster=w291, "Results Data Array"=w287) -> (w290:T5)
        n106 = call <vilib>:"Add State(s) to Queue__jki_lib_state_machine.vi"("State(s) in (\"\")"=w299) -> ("States Out"=w298:string)  [unwired: 14 in]
      }
      frame "---------- Results Data ----------" {
        # "Template Separator\n(You can make a copy of, or modify, this frame)"
        n107 = call <vilib>:"Add State(s) to Queue__jki_lib_state_machine.vi"("State(s) in (\"\")"=w303) -> ("States Out"=w302:string)  [unwired: 14 in]
      }
      frame "Results Data: Write Results Data" {
        w305 = ","  # delimiter (\t)
        w306 = TRUE  # append to file? (new file:F)
        n108 = Unbundle By Name(w308) -> ("Results File Path"=w307:path, "Results Data Array"=w304:string[][])
        "Results Data Array" <- w304
        n109 = call-poly <vilib>:"Write Delimited Spreadsheet.vi"("file path (dialog if empty)"=w307, "2D data"=w304, "append to file? (new file:F)"=w306, "error in (no error)"=w309, "delimiter (\\t)"=w305) -> ("error out"=w310:errorcluster)  [unwired: 9 in, 1 out]
        n110 = call <vilib>:"Add State(s) to Queue__jki_lib_state_machine.vi"("State(s) in (\"\")"=w312) -> ("States Out"=w311:string)  [unwired: 14 in]
      }
      frame "---------- Fuse 5 ----------" {
        # "Template Separator\n(You can make a copy of, or modify, this frame)"
        n111 = call <vilib>:"Add State(s) to Queue__jki_lib_state_machine.vi"("State(s) in (\"\")"=w316) -> ("States Out"=w315:string)  [unwired: 14 in]
      }
      frame "Fuse 5: Initialise" {
        # "Measurement initialisation code goes here"
        n112 = call "FGV - Initialise.vi"("Enum"=FGV_-_Enum."Get Data", "Error In"=w321) -> ("connection ID"=w318:refnum<k16>, "Handle Out"=w317:u64, "Error Out"=w320:errorcluster)  [unwired: 13 in, 2 out]
        n113 = Bundle By Name(cluster=w323, "connection ID"=w318, "handle out"=w317) -> (w322:T5)
        n114 = call <vilib>:"Add State(s) to Queue__jki_lib_state_machine.vi"("State(s) in (\"\")"=w325) -> ("States Out"=w324:string)  [unwired: 14 in]
      }
      frame "Fuse 5: Start Timer" {
        # "Start Timer and slide bar"
        # "Template Separator\n(You can make a copy of, or modify, this frame)"
        n115 = call "Timer.vi"("error in (no error)"=w327, "Enum"=T4."Start Timer") -> ("error out"=w331:errorcluster)  [unwired: 6 in, 3 out]
        n116 = property on="Timeout - Test" class="Slide (strict)"(error in=w331, "Value"=0.0 ("Horizontal Pointer Slide"), "Scale.Maximum"=5.0 ("Target Time"), "Scale.Minimum"=0.0 ("Scale.Range:Minimum")) -> (error out=w326:errorcluster)  [unwired: 1 in, 1 out]
        n117 = call <vilib>:"Add State(s) to Queue__jki_lib_state_machine.vi"("State(s) in (\"\")"=w335) -> ("States Out"=w334:string)  [unwired: 14 in]
      }
      frame "Fuse 5: I2C Measurment" {
        # "switch realy - trigger estop 1"
        n118 = Unbundle By Name(w342) -> ("handle out"=w337:u64)
        n119 = call "PCA9525 - CJB.vi"("error in (no error)"=w340, "buffer"=u8[] [2, 16, 22], "handle"=w337) -> ("error out"=w339:errorcluster, "handle out"=w338:u64)  [unwired: 7 in]
        n120 = Bundle By Name(cluster=w342, "handle out"=w338) -> (w341:T5)
        n121 = call <vilib>:"Add State(s) to Queue__jki_lib_state_machine.vi"("State(s) in (\"\")"=w344) -> ("States Out"=w343:string)  [unwired: 14 in]
      }
      frame "Fuse 5: UDP Read" {
        # "Read UDP if equal to F1 then test complete if false timer is check if elapsed"
        n122 = Unbundle By Name(w356) -> ("connection ID"=w364:refnum<k16>)
        n123 = UDP Read(connection ID=w364, timeout ms (25000)=1, 8:w357) -> (data out=w351:string, error out=w355:errorcluster, 3:w363:refnum<k16>)  [unwired: 1 in, 2 out]
        n124 = String Subset(string=w351, offset (0)=93 ("offset (0) 2"), length (rest)=3 ("length (rest) 2")) -> (substring=w362:string)
        n125 = String To Byte Array(string=w362) -> (unsigned byte array=w369:u8[])
        n126 = Number To Hexadecimal String(1:i16 2 ("width (-)"), 2:w369) -> (0:w368:string[])
        n127 = Index Array(array=w368, index #1=0 ("index")) -> (element #1=w349:string, element #2=w348:string, element #3=w347:string)  [unwired: 2 in]
        n128 = Concatenate Strings(w349, w348, w347) -> (w346:string)
        n129 = call <vilib>:"Clear Errors.vi"("error in (no error)"=w355, "specific error code to clear (0: all)"=56) -> ("error out"=w354:errorcluster)  [unwired: 4 in, 1 out]
        n130 = Equal?(x=w346, y="0004C3") -> (x = y?=w350:bool)
        "Fuse 5 Test" <- w350
        n131 = Bundle By Name(cluster=w356, "connection ID"=w363, "Fuse 5 Test"=w346) -> (w370:T5)
        n132 = call-poly <vilib>:"Select State(s)__jki_lib_state_machine.vi"("State(s) if True (\"\")"="Macro: Test (2)" ("State(s) if True (\"\")"), "Select"=w350, "State(s) if False (\"\")"="Fuse 5: Elapsed Timer" ("State(s) if False (\"\")")) -> ("States Out"=w358:string)  [unwired: 12 in]
        n133 = call <vilib>:"Add State(s) to Queue__jki_lib_state_machine.vi"("State(s) in Front (\"\")"=w358, "State(s) in (\"\")"=w372) -> ("States Out"=w371:string)  [unwired: 13 in]
      }
      frame "Fuse 5: Elapsed Timer" {
        # "check if timer elapsed if true end of test if false UDP is read again,"
        # "Template Separator\n(You can make a copy of, or modify, this frame)"
        n134 = call "Timer.vi"("error in (no error)"=w377, "Target Time"=5.0, "Enum"=T4."Get Time") -> ("error out"=w376:errorcluster, "Time Elapsed?"=w378:bool, "Elapsed Time"=→"Timeout - Test":dbl)  [unwired: 5 in, 1 out]
        n135 = call-poly <vilib>:"Select State(s)__jki_lib_state_machine.vi"("State(s) if True (\"\")"="Macro: Test (2)" ("State(s) if True (\"\")"), "Select"=w378, "State(s) if False (\"\")"="Fuse 5: UDP Read" ("State(s) if False (\"\")")) -> ("States Out"=w375:string)  [unwired: 12 in]
        n136 = call <vilib>:"Add State(s) to Queue__jki_lib_state_machine.vi"("State(s) in Front (\"\")"=w375, "State(s) in (\"\")"=w384) -> ("States Out"=w383:string)  [unwired: 13 in]
      }
      frame "Fuse 5: Start Timer (State)" {
        # "Start Timer and slide bar"
        # "Template Separator\n(You can make a copy of, or modify, this frame)"
        n137 = call "Timer.vi"("error in (no error)"=w386, "Enum"=T4."Start Timer") -> ("error out"=w390:errorcluster)  [unwired: 6 in, 3 out]
        n138 = property on="Timeout - Test 2" class="Slide (strict)"(error in=w390, "Value"=0.0 ("Horizontal Pointer Slide"), "Scale.Maximum"=10.0 ("Target Time"), "Scale.Minimum"=0.0 ("Scale.Range:Minimum")) -> (error out=w385:errorcluster)  [unwired: 1 in, 1 out]
        n139 = call <vilib>:"Add State(s) to Queue__jki_lib_state_machine.vi"("State(s) in (\"\")"=w394) -> ("States Out"=w393:string)  [unwired: 14 in]
      }
      frame "Fuse 5: UDP Read (State)" {
        # "Read UDP if equal to F1 then test complete if false timer is check if elapsed"
        n140 = Unbundle By Name(w405) -> ("connection ID"=w410:refnum<k16>)
        n141 = UDP Read(connection ID=w410, timeout ms (25000)=1, 8:w399) -> (data out=w400:string, error out=w404:errorcluster, 3:w409:refnum<k16>)  [unwired: 1 in, 2 out]
        n142 = String Subset(string=w400, offset (0)=17 ("offset (0) 2"), length (rest)=1 ("length (rest) 2")) -> (substring=w408:string)
        n143 = String To Byte Array(string=w408) -> (unsigned byte array=w415:u8[])
        n144 = Number To Hexadecimal String(2:w415) -> (0:w414:string[])  [unwired: 1 in]
        n145 = Index Array(array=w414, index=0) -> (element=w406:string)
        n146 = Equal?(x=w406, y="19") -> (x = y?=w396:bool)
        "State Test" <- w396
        n147 = Bundle By Name(cluster=w405, "connection ID"=w409, "Fuse 5 State Test"=w406) -> (w416:T5)
        n148 = call <vilib>:"Clear Errors.vi"("error in (no error)"=w404, "specific error code to clear (0: all)"=56) -> ("error out"=w403:errorcluster)  [unwired: 4 in, 1 out]
        n149 = call-poly <vilib>:"Select State(s)__jki_lib_state_machine.vi"("State(s) if True (\"\")"="Macro: Limits" ("State(s) if True (\"\")"), "Select"=w396, "State(s) if False (\"\")"="Fuse 5: Elapsed Timer (State)" ("State(s) if False (\"\")")) -> ("States Out"=w395:string)  [unwired: 12 in]
        n150 = call <vilib>:"Add State(s) to Queue__jki_lib_state_machine.vi"("State(s) in Front (\"\")"=w395, "State(s) in (\"\")"=w418) -> ("States Out"=w417:string)  [unwired: 13 in]
      }
      frame "Fuse 5: Elapsed Timer (State)" {
        # "check if timer elapsed if true end of test if false UDP is read again,"
        # "Template Separator\n(You can make a copy of, or modify, this frame)"
        n151 = call "Timer.vi"("error in (no error)"=w423, "Target Time"=10.0, "Enum"=T4."Get Time") -> ("error out"=w422:errorcluster, "Time Elapsed?"=w424:bool, "Elapsed Time"=→"Timeout - Test 2":dbl)  [unwired: 5 in, 1 out]
        n152 = call-poly <vilib>:"Select State(s)__jki_lib_state_machine.vi"("State(s) if True (\"\")"="Macro: Limits" ("State(s) if True (\"\")"), "Select"=w424, "State(s) if False (\"\")"="Fuse 5: UDP Read (State)" ("State(s) if False (\"\")")) -> ("States Out"=w421:string)  [unwired: 12 in]
        n153 = call <vilib>:"Add State(s) to Queue__jki_lib_state_machine.vi"("State(s) in Front (\"\")"=w421, "State(s) in (\"\")"=w430) -> ("States Out"=w429:string)  [unwired: 13 in]
      }
    }
    n154 = Wait (ms)(milliseconds to wait=u32 0) -> ()  [unwired: 1 out]
  }
  "error out" <- w1
